vi "Autonomous Independent.vi"() -> ()   [LabVIEW 2017]
doc: "This VI is called when autonomous begins, and will automatically be terminated when autonomous ends. You can carry out timed or sensor driven robot movement independently without needing to return to the caller."
uses:
  Auto/Auto switch direita.ctl
  LabVIEW_is_Under_Control.lib/Util/Unpack Gamepad/Button Cluster.ctl
  Robot Global Data.vi
  <vilib>/Rock Robotics/Network Tables/NT Read String.vi
panel:
  out "auto state":T1=enum."Girando"
  in  "DistanceAfterTurn2":dbl
  in  "DistanciaSwitch 2":dbl
  in  "Setpoint(degrees) 2":dbl=90.0 format="%#_13g"
  in  "Setpoint(degrees)":dbl=-90.0 format="%#_13g"
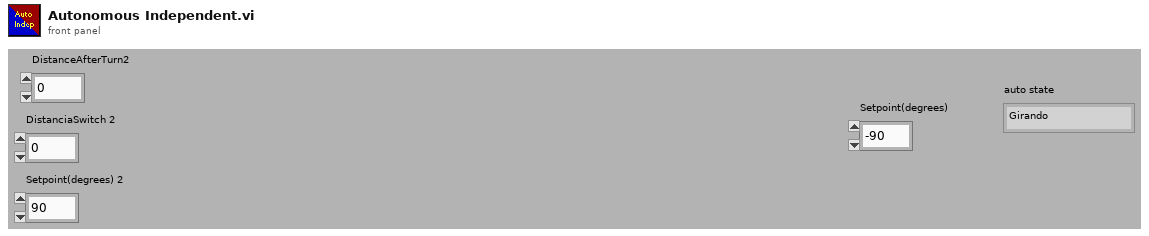
[diagram p1: front panel]
types:
  T1 = typedef "Auto switch direita.ctl" = enum16{"Zerandosensor", "Girando", "Andando", "Jogando", "Andando2", "Finalizando", "Zerandosensor2"}
  T2 = cluster{"proportional gain (Kc)":dbl, "integral time (Ti, min)":dbl, "derivative time (Td, min)":dbl}
  T3 = typedef "Button Cluster.ctl" = cluster{"Buttons[0]":bool, "Buttons[1]":bool, "Buttons[2]":bool, "Buttons[3]":bool, "Buttons[4]":bool, "Buttons[5]":bool, "Buttons[6]":bool, "Buttons[7]":bool, "Buttons[8]":bool, "Buttons[9]":bool}
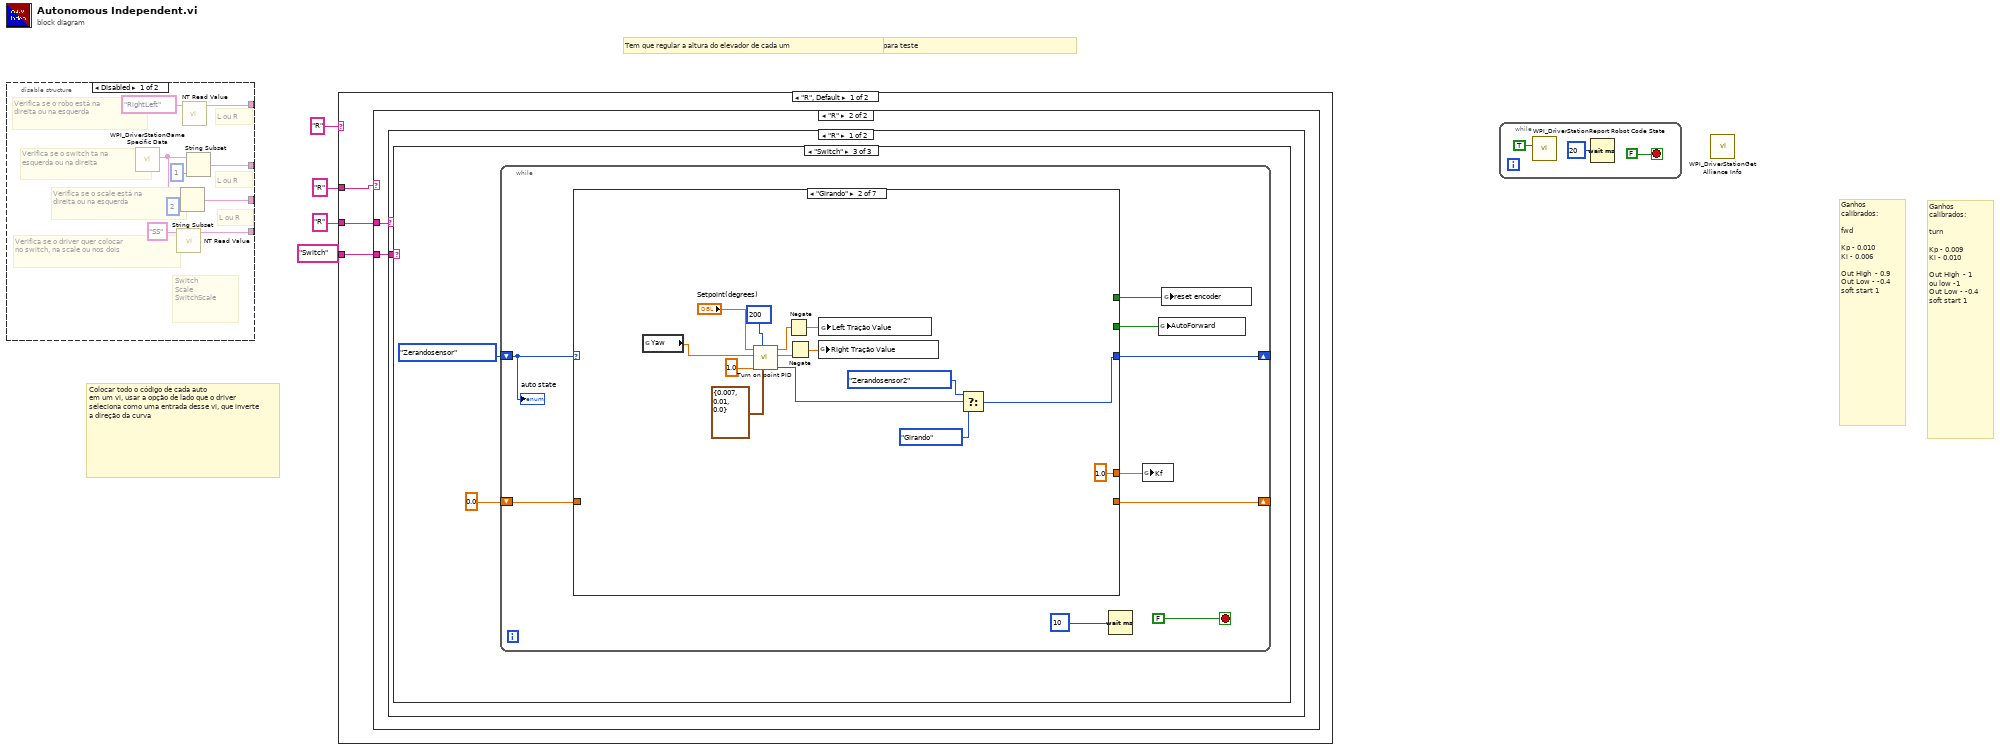
[diagram p0: block diagram]
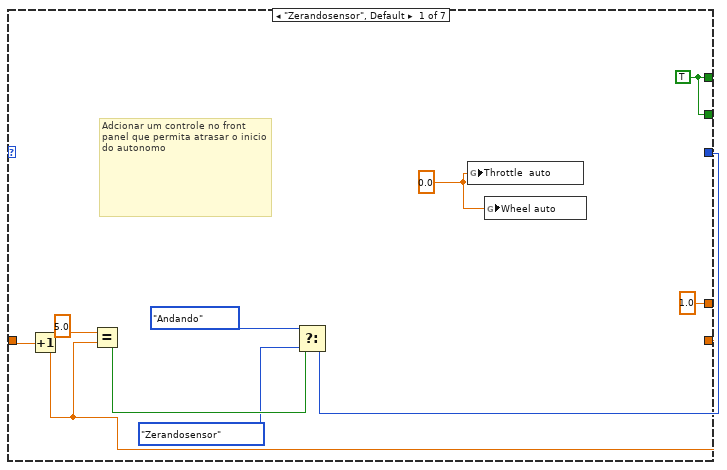
[diagram p9: hidden frame]
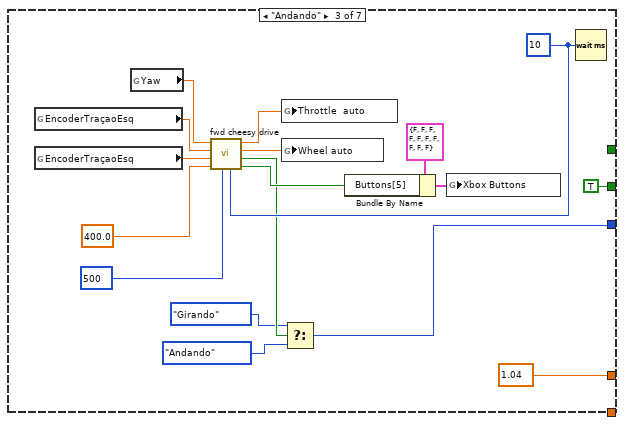
[diagram p10: hidden frame]
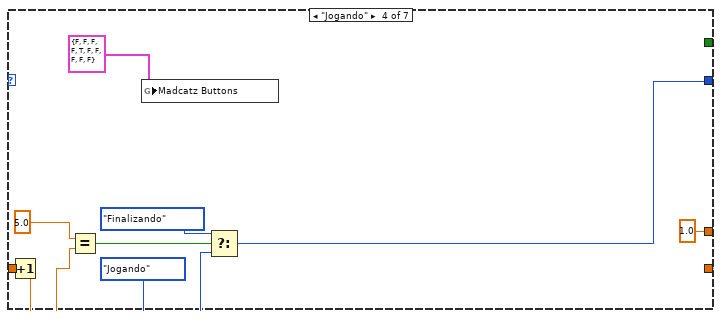
[diagram p11: hidden frame]
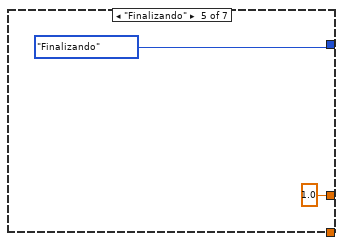
[diagram p12: hidden frame]
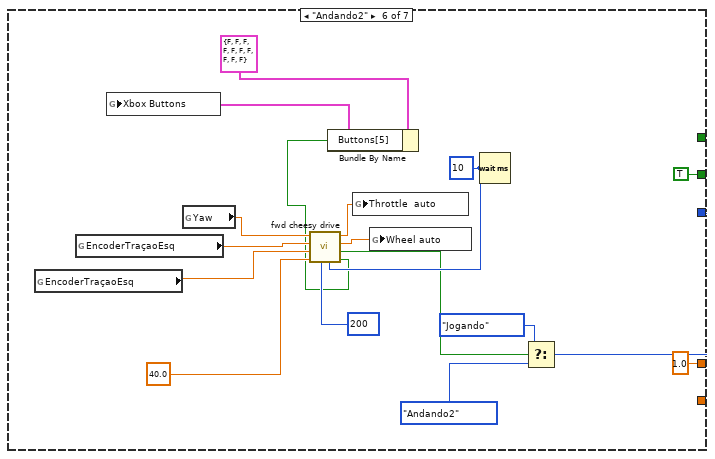
[diagram p13: hidden frame]
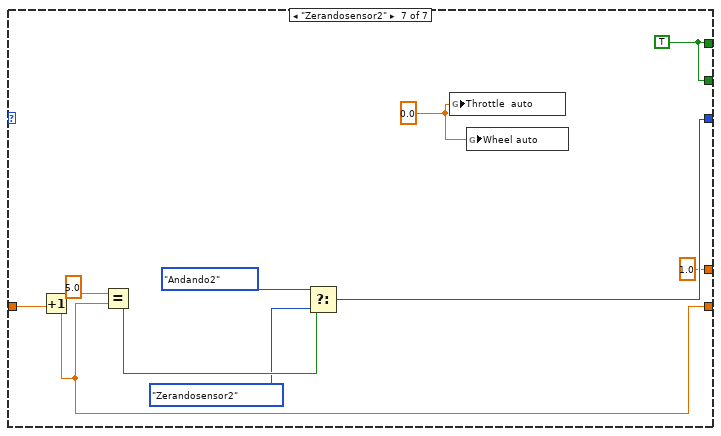
[diagram p14: hidden frame]
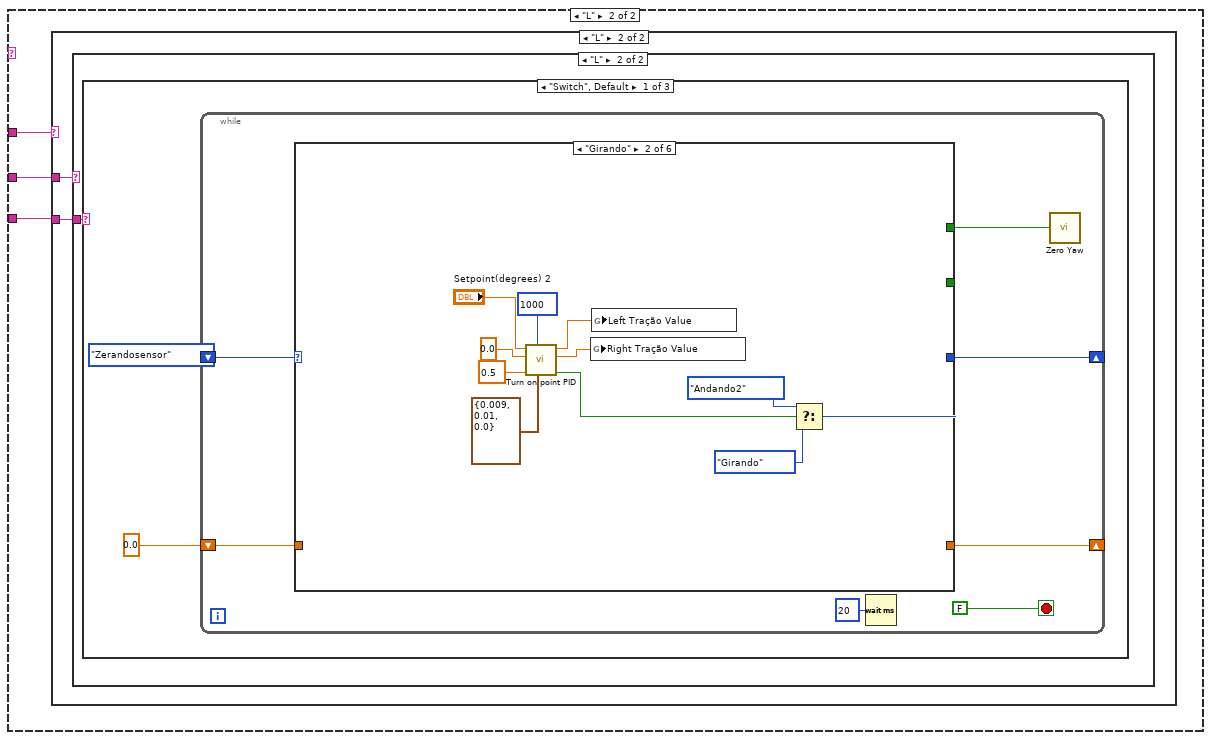
[diagram p17: hidden frame]
diagram:
  # "Colocar todo o código de cada auto\nem um vi, usar a opção de lado que o driver seleciona como uma entrada desse vi, que inverte a direção da curva"
  # "Tem que regular a altura do elevador de cada um"
  # "Tem que regular a distancia de cada quadrado quando a pista estiver pronta para teste"
  # "Ganhos calibrados:\n\nturn\n\nKp - 0.009\nKi - 0.010\n\nOut High  - 1\nou low -1\nOut Low - -0.4\nsoft start 1"
  # "Ganhos calibrados:\n\nfwd\n\nKp - 0.010\nKi - 0.006\n\nOut High  - 0.9\nOut Low - -0.4\nsoft start 1"
  n1 = disable-structure shown="Disabled" {
    disable-tunnel: [w12 _] -> _
    disable-tunnel: [w10 _] -> _
    disable-tunnel: [w7 _] -> _
    disable-tunnel: [w5 _] -> _
    frame Disabled {
      # "Switch\nScale\nSwitchScale"
      # "L ou R"
      # "L ou R"
      # "L ou R"
      # "Verifica se o driver quer colocar\nno switch, na scale ou nos dois"
      # "Verifica se o scale está na\ndireita ou na esquerda"
      # "Verifica se o switch ta na\nesquerda ou na direita"
      # "Verifica se o robo está na\ndireita ou na esquerda"
      n2 = call <vilib>:"WPI_DriverStationGame Specific Data.vi"() -> ("Game Specific Data"=w8:string)  [unwired: 11 in]
      n3 = call-poly <vilib>:"NT Read Value.vi"("Name"="SS") -> ("String"=w5:string)  [unwired: 9 in, 1 out]
      n4 = String Subset(string=w8, length (rest)=2 ("length (rest)")) -> (substring=w7:string)  [unwired: 1 in]
      n5 = call-poly <vilib>:"NT Read Value.vi"("Name"="RightLeft") -> ("String"=w12:string)  [unwired: 9 in, 1 out]
      n6 = String Subset(string=w8, length (rest)=1 ("length (rest)")) -> (substring=w10:string)  [unwired: 1 in]
    }
    frame Enabled {
    }
  }
  n7 = case shown="\"R\", Default" "R" {
    tunnel: "R" -> [w16 w117]
    tunnel: "R" -> [w15 w116]
    tunnel: "Switch" -> [w14 w115]
    frame "R", Default {
      n8 = case shown="\"R\"" w16 {
        tunnel: w15 -> [w18 w22]
        tunnel: w14 -> [w17 w21]
        frame "L", Default {
          n9 = case shown="\"R\", Default" w18 {
            tunnel: w17 -> [w19 w20]
            frame "R", Default {
              n10 = case shown="\"Scale\"" w19 {
                frame "Switch", Default {
                }
                frame "Scale" {
                }
              }
            }
            frame "L" {
              n11 = case shown="\"Scale\", Default" w20 {
                frame "Scale", Default {
                }
                frame "Switch" {
                }
              }
            }
          }
        }
        frame "R" {
          n12 = case shown="\"R\"" w22 {
            tunnel: w21 -> [w23 w114]
            frame "R" {
              n13 = case shown="\"Switch\"" w23 {
                frame "Scale", Default {
                }
                frame "SwitchScale" {
                }
                frame "Switch" {
                  n14 = while {
                    shift-right: [w30] -> _
                    shift-left: Auto_switch_direita."Zerandosensor" -> [w28]
                    shift-right: [w31] -> _
                    shift-left: 0.0 -> [w32]
                    stop <- FALSE stop-if-true
                    n15 = case shown="\"Girando\"" w28 {
                      tunnel: w32 -> [w44 _ _ w83 _ _ w105]
                      tunnel: [w41 _ _ w80 _ _ w106] -> w31
                      tunnel: [w40 w55 w63 w79 Auto_switch_direita."Finalizando" w89 w107] -> w30
                      tunnel: [w37 _ _ _ _ _ w112] -> w27
                      tunnel: [w37 _ TRUE _ _ TRUE w112] -> w29
                      tunnel: [1.0 1.0 1.04 1.0 1.0 1.0 1.0] -> w26
                      frame "Zerandosensor", Default {
                        w36 = 0.0
                        w37 = TRUE
                        # "Adcionar um controle no front panel que permita atrasar o inicio do autonomo"
                        n16 = Increment(x=w44) -> (x+1=w41:dbl)
                        n17 = Equal?(x=5.0, y=w41) -> (x = y?=w42:bool)
                        n18 = Select(t=Auto_switch_direita."Andando", s=w42, f=Auto_switch_direita."Zerandosensor") -> (s? t:f=w40:T1)
                        n19 = global write "Robot Global Data.vi" "Throttle  auto"(w36) -> ()
                        n20 = global write "Robot Global Data.vi" "Wheel auto"(w36) -> ()
                      }
                      frame "Girando" {
                        n21 = global read "Robot Global Data.vi" "Yaw"() -> (w48:dbl)
                        n22 = call "Turn on point PID.vi"("Gains"=T2 {"proportional gain (Kc)"=0.007, "integral time (Ti, min)"=0.01, "derivative time (Td, min)"=0.0}, "Time to stop"=200, "Precision"=1.0, "Yaw"=w48, "Setpoint(degrees)"="Setpoint(degrees)") -> ("Finished?"=w56:bool, "PWM right"=w51:dbl, "PWM left"=w52:dbl)  [unwired: 4 in]
                        n23 = Negate(x=w52) -> (-x=w47:dbl)
                        n24 = Negate(x=w51) -> (-x=w46:dbl)
                        n25 = global write "Robot Global Data.vi" "Right Tração Value"(w46) -> ()
                        n26 = global write "Robot Global Data.vi" "Left Tração Value"(w47) -> ()
                        n27 = Select(t=Auto_switch_direita."Zerandosensor2", s=w56, f=Auto_switch_direita."Girando") -> (s? t:f=w55:T1)
                      }
                      frame "Andando" {
                        w71 = u32 10 ("milliseconds to wait")
                        n28 = global read "Robot Global Data.vi" "EncoderTraçaoEsq"() -> (w73:dbl)
                        n29 = global read "Robot Global Data.vi" "EncoderTraçaoEsq"() -> (w74:dbl)
                        n30 = global read "Robot Global Data.vi" "Yaw"() -> (w75:dbl)
                        n31 = call "fwd cheesy drive.vi"("Loop Timer"=w71, "Time to stop"=500, "Distance"=400.0 ("DistanceSwitch"), "Encoder Left"=w74, "Encoder Right"=w73, "Yaw"=w75) -> ("Finished distance"=w65:bool, "Both finished"=w64:bool, "Direction"=w69:dbl, "Trottle"=w68:dbl)  [unwired: 2 in]
                        n32 = global write "Robot Global Data.vi" "Throttle  auto"(w68) -> ()
                        n33 = global write "Robot Global Data.vi" "Wheel auto"(w69) -> ()
                        n34 = Select(t=Auto_switch_direita."Girando", s=w64, f=Auto_switch_direita."Andando") -> (s? t:f=w63:T1)
                        n35 = Bundle By Name(cluster=T3 {"Buttons[0]"=FALSE, "Buttons[1]"=FALSE, "Buttons[2]"=FALSE, "Buttons[3]"=FALSE, "Buttons[4]"=FALSE, "Buttons[5]"=FALSE, "Buttons[6]"=FALSE, "Buttons[7]"=FALSE, "Buttons[8]"=FALSE, "Buttons[9]"=FALSE} ("Xbox Buttons"), "Buttons[5]"=w65) -> (w66:T3)
                        n36 = global write "Robot Global Data.vi" "Xbox Buttons"(w66) -> ()
                        n37 = Wait (ms)(milliseconds to wait=w71) -> ()  [unwired: 1 out]
                      }
                      frame "Jogando" {
                        n38 = Increment(x=w83) -> (x+1=w80:dbl)
                        n39 = Equal?(x=5.0, y=w80) -> (x = y?=w81:bool)
                        n40 = global write "Robot Global Data.vi" "Madcatz Buttons"(T3 {"Buttons[0]"=FALSE, "Buttons[1]"=FALSE, "Buttons[2]"=FALSE, "Buttons[3]"=FALSE, "Buttons[4]"=TRUE, "Buttons[5]"=FALSE, "Buttons[6]"=FALSE, "Buttons[7]"=FALSE, "Buttons[8]"=FALSE, "Buttons[9]"=FALSE} ("Madcatz Buttons")) -> ()
                        n41 = Select(t=Auto_switch_direita."Finalizando", s=w81, f=Auto_switch_direita."Jogando") -> (s? t:f=w79:T1)
                      }
                      frame "Finalizando" {
                      }
                      frame "Andando2" {
                        w99 = u32 10 ("milliseconds to wait")
                        n42 = global read "Robot Global Data.vi" "EncoderTraçaoEsq"() -> (w102:dbl)
                        n43 = global read "Robot Global Data.vi" "EncoderTraçaoEsq"() -> (w101:dbl)
                        n44 = global read "Robot Global Data.vi" "Yaw"() -> (w103:dbl)
                        n45 = call "fwd cheesy drive.vi"("Loop Timer"=w99, "Time to stop"=200, "Distance"=40.0 ("DistanceAfterTurn"), "Encoder Left"=w102, "Encoder Right"=w101, "Yaw"=w103) -> ("Finished distance"=w93:bool, "Both finished"=w92:bool, "Direction"=w97:dbl, "Trottle"=w96:dbl)  [unwired: 2 in]
                        n46 = Bundle By Name(cluster=T3 {"Buttons[0]"=FALSE, "Buttons[1]"=FALSE, "Buttons[2]"=FALSE, "Buttons[3]"=FALSE, "Buttons[4]"=FALSE, "Buttons[5]"=FALSE, "Buttons[6]"=FALSE, "Buttons[7]"=FALSE, "Buttons[8]"=FALSE, "Buttons[9]"=FALSE} ("Xbox Buttons"), "Buttons[5]"=w93) -> (w94:T3)
                        n47 = global write "Robot Global Data.vi" "Xbox Buttons"(w94) -> ()
                        n48 = global write "Robot Global Data.vi" "Throttle  auto"(w96) -> ()
                        n49 = global write "Robot Global Data.vi" "Wheel auto"(w97) -> ()
                        n50 = Wait (ms)(milliseconds to wait=w99) -> ()  [unwired: 1 out]
                        n51 = Select(t=Auto_switch_direita."Jogando", s=w92, f=Auto_switch_direita."Andando2") -> (s? t:f=w89:T1)
                      }
                      frame "Zerandosensor2" {
                        w112 = TRUE
                        w113 = 0.0
                        n52 = Increment(x=w105) -> (x+1=w106:dbl)
                        n53 = Equal?(x=5.0, y=w106) -> (x = y?=w110:bool)
                        n54 = Select(t=Auto_switch_direita."Andando2", s=w110, f=Auto_switch_direita."Zerandosensor2") -> (s? t:f=w107:T1)
                        n55 = global write "Robot Global Data.vi" "Throttle  auto"(w113) -> ()
                        n56 = global write "Robot Global Data.vi" "Wheel auto"(w113) -> ()
                      }
                    }
                    n57 = Wait (ms)(milliseconds to wait=u32 10) -> ()  [unwired: 1 out]
                    n58 = global write "Robot Global Data.vi" "Kf"(w26) -> ()
                    n59 = global write "Robot Global Data.vi" "AutoForward"(w29) -> ()
                    n60 = global write "Robot Global Data.vi" "reset encoder"(w27) -> ()
                    "auto state" <- w28
                  }
                }
              }
            }
            frame "L", Default {
              n61 = case shown="\"Switch\"" w114 {
                frame "Scale", Default {
                }
                frame "Switch" {
                }
              }
            }
          }
        }
      }
    }
    frame "L" {
      n62 = case shown="\"L\"" w117 {
        tunnel: w116 -> [w119 w123]
        tunnel: w115 -> [w118 w122]
        frame "R", Default {
          n63 = case shown="\"R\", Default" w119 {
            tunnel: w118 -> [w120 w121]
            frame "R", Default {
              n64 = case shown="\"Scale\"" w120 {
                frame "Switch", Default {
                }
                frame "Scale" {
                }
              }
            }
            frame "L" {
              n65 = case shown="\"Switch\", Default" w121 {
                frame "Switch", Default {
                }
                frame "Scale" {
                }
              }
            }
          }
        }
        frame "L" {
          n66 = case shown="\"L\"" w123 {
            tunnel: w122 -> [w124 w125]
            frame "R", Default {
              n67 = case shown="\"Scale\", Default" w124 {
                frame "Scale", Default {
                }
                frame "Switch" {
                }
              }
            }
            frame "L" {
              n68 = case shown="\"Switch\", Default" w125 {
                frame "Switch", Default {
                  n69 = while {
                    shift-right: [w129] -> _
                    shift-left: Auto_switch_direita."Zerandosensor" -> [w133]
                    shift-right: [w130] -> _
                    shift-left: 0.0 -> [w131]
                    stop <- FALSE stop-if-true
                    n70 = case shown="\"Girando\"" w133 {
                      tunnel: w131 -> [w143 _ _ w176 _ _]
                      tunnel: [w140 _ _ w173 _ _] -> w130
                      tunnel: [w139 w150 w157 w172 Auto_switch_direita."Finalizando" w179] -> w129
                      tunnel: [TRUE _ _ _ _ _] -> w128
                      tunnel: [TRUE _ _ _ _ _] -> _
                      frame "Zerandosensor", Default {
                        n71 = Increment(x=w143) -> (x+1=w140:dbl)
                        n72 = Equal?(x=5.0, y=w140) -> (x = y?=w141:bool)
                        n73 = Select(t=Auto_switch_direita."Andando", s=w141, f=Auto_switch_direita."Zerandosensor") -> (s? t:f=w139:T1)
                      }
                      frame "Girando" {
                        n74 = call "Turn on point PID.vi"("Gains"=T2 {"proportional gain (Kc)"=0.009, "integral time (Ti, min)"=0.01, "derivative time (Td, min)"=0.0}, "Time to stop"=1000, "Precision"=0.5, "Yaw"=0.0, "Setpoint(degrees)"="Setpoint(degrees) 2") -> ("Finished?"=w151:bool, "PWM right"=w146:dbl, "PWM left"=w147:dbl)  [unwired: 4 in]
                        n75 = global write "Robot Global Data.vi" "Right Tração Value"(w146) -> ()
                        n76 = global write "Robot Global Data.vi" "Left Tração Value"(w147) -> ()
                        n77 = Select(t=Auto_switch_direita."Andando2", s=w151, f=Auto_switch_direita."Girando") -> (s? t:f=w150:T1)
                      }
                      frame "Andando" {
                        w165 = u32 10 ("milliseconds to wait")
                        n78 = global read "Robot Global Data.vi" "EncoderTraçaoEsq"() -> (w167:dbl)
                        n79 = global read "Robot Global Data.vi" "EncoderTraçaoEsq"() -> (w168:dbl)
                        n80 = global read "Robot Global Data.vi" "Yaw"() -> (w169:dbl)
                        n81 = call "fwd cheesy drive.vi"("Loop Timer"=w165, "Time to stop"=1000, "Distance"="DistanciaSwitch 2", "Encoder Left"=w168, "Encoder Right"=w167, "Yaw"=w169) -> ("Finished distance"=w159:bool, "Both finished"=w158:bool, "Direction"=w163:dbl, "Trottle"=w162:dbl)  [unwired: 2 in]
                        n82 = Bundle By Name(cluster=T3 {"Buttons[0]"=FALSE, "Buttons[1]"=FALSE, "Buttons[2]"=FALSE, "Buttons[3]"=FALSE, "Buttons[4]"=FALSE, "Buttons[5]"=FALSE, "Buttons[6]"=FALSE, "Buttons[7]"=FALSE, "Buttons[8]"=FALSE, "Buttons[9]"=FALSE} ("Xbox Buttons"), "Buttons[5]"=w159) -> (w160:T3)
                        n83 = global write "Robot Global Data.vi" "Throttle  auto"(w162) -> ()
                        n84 = global write "Robot Global Data.vi" "Xbox Buttons"(w160) -> ()
                        n85 = global write "Robot Global Data.vi" "Wheel auto"(w163) -> ()
                        n86 = Wait (ms)(milliseconds to wait=w165) -> ()  [unwired: 1 out]
                        n87 = Select(t=Auto_switch_direita."Girando", s=w158, f=Auto_switch_direita."Andando") -> (s? t:f=w157:T1)
                      }
                      frame "Jogando" {
                        n88 = Increment(x=w176) -> (x+1=w173:dbl)
                        n89 = Equal?(x=5.0, y=w173) -> (x = y?=w174:bool)
                        n90 = global write "Robot Global Data.vi" "Madcatz Buttons"(T3 {"Buttons[0]"=FALSE, "Buttons[1]"=FALSE, "Buttons[2]"=FALSE, "Buttons[3]"=FALSE, "Buttons[4]"=TRUE, "Buttons[5]"=FALSE, "Buttons[6]"=FALSE, "Buttons[7]"=FALSE, "Buttons[8]"=FALSE, "Buttons[9]"=FALSE} ("Madcatz Buttons")) -> ()
                        n91 = Select(t=Auto_switch_direita."Finalizando", s=w174, f=Auto_switch_direita."Jogando") -> (s? t:f=w172:T1)
                      }
                      frame "Finalizando" {
                      }
                      frame "Andando2" {
                        w189 = u32 10 ("milliseconds to wait")
                        n92 = global read "Robot Global Data.vi" "EncoderTraçaoEsq"() -> (w191:dbl)
                        n93 = global read "Robot Global Data.vi" "EncoderTraçaoEsq"() -> (w192:dbl)
                        n94 = global read "Robot Global Data.vi" "Yaw"() -> (w193:dbl)
                        n95 = call "fwd cheesy drive.vi"("Loop Timer"=w189, "Time to stop"=1000, "Distance"="DistanceAfterTurn2", "Encoder Left"=w192, "Encoder Right"=w191, "Yaw"=w193) -> ("Finished distance"=w183:bool, "Both finished"=w182:bool, "Direction"=w187:dbl, "Trottle"=w186:dbl)  [unwired: 2 in]
                        n96 = Bundle By Name(cluster=T3 {"Buttons[0]"=FALSE, "Buttons[1]"=FALSE, "Buttons[2]"=FALSE, "Buttons[3]"=FALSE, "Buttons[4]"=FALSE, "Buttons[5]"=FALSE, "Buttons[6]"=FALSE, "Buttons[7]"=FALSE, "Buttons[8]"=FALSE, "Buttons[9]"=FALSE} ("Xbox Buttons"), "Buttons[5]"=w183) -> (w184:T3)
                        n97 = global write "Robot Global Data.vi" "Throttle  auto"(w186) -> ()
                        n98 = global write "Robot Global Data.vi" "Xbox Buttons"(w184) -> ()
                        n99 = global write "Robot Global Data.vi" "Wheel auto"(w187) -> ()
                        n100 = Wait (ms)(milliseconds to wait=w189) -> ()  [unwired: 1 out]
                        n101 = Select(t=Auto_switch_direita."Jogando", s=w182, f=Auto_switch_direita."Andando2") -> (s? t:f=w179:T1)
                      }
                    }
                    n102 = Wait (ms)(milliseconds to wait=u32 20) -> ()  [unwired: 1 out]
                    n103 = call <vilib>:"Zero Yaw.vi"("Zero"=w128) -> ()  [unwired: 11 in]
                  }
                }
                frame "Scale" {
                }
                frame "SwitchScale" {
                }
              }
            }
          }
        }
      }
    }
  }
  n104 = while {
    stop <- FALSE stop-if-true
    n105 = call <vilib>:"WPI_DriverStationReport Robot Code State.vi"("Autonomous"=TRUE) -> ()  [unwired: 10 in, 1 out]
    n106 = Wait (ms)(milliseconds to wait=u32 20) -> ()  [unwired: 1 out]
  }
  n107 = call <vilib>:"WPI_DriverStationGet Alliance Info.vi"() -> ()  [unwired: 12 out]
